vi "Temperature Response.vi"(8 "error in (no error)":errorcluster, 9 "Diagnostics":string, 10 "Sender":string, 11 "Pulse Controller in":refnum<class "Pulse Controller.lvclass">) -> (0 "error out":errorcluster, 3 "Pulse Controller out":refnum<class "Pulse Controller.lvclass">)   [LabVIEW 2024, in "Pulse Controller.lvclass"]
uses:
  Pulse Controller.lvclass
  Pulse Controller.lvclass/Pulse Controller.ctl
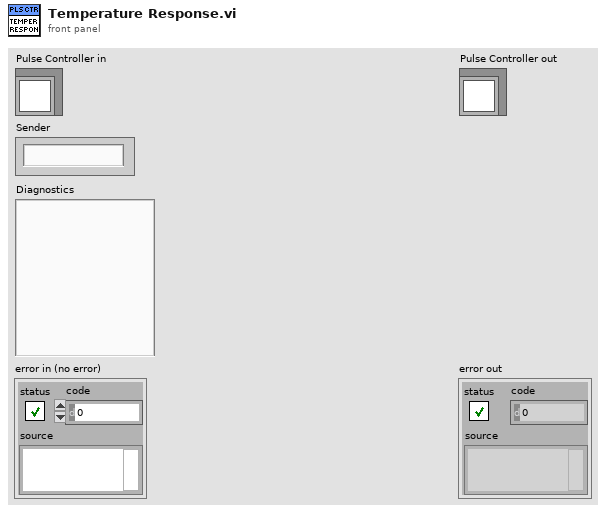
[diagram p1: front panel]
types:
  T1 = typedef "Worker State.ctl" = enum16{"Idle", "Starting", "Working", "Stopping"}
  T2 = cluster{"seconds since 1Jan1904":timestamp, "Sender":string, "Diagnostics":string}
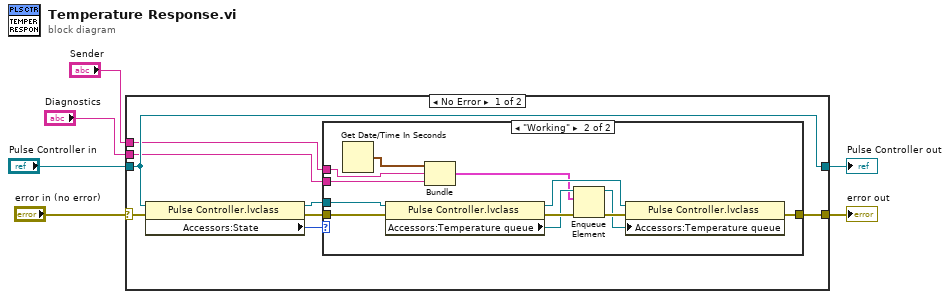
[diagram p0: block diagram]
diagram:
  n1 = case shown="No Error" "error in (no error)" {
    selector: "error in (no error)" -> [w12 w29]
    tunnel: [w11 w29] -> w5
    tunnel: [w14 w28] -> w3
    tunnel: "Pulse Controller in" -> [w14 w28]
    tunnel: "Diagnostics" -> [w9 _]
    tunnel: "Sender" -> [w8 _]
    frame No Error {
      n2 = property class="Pulse Controller.lvclass"(reference=w14, error in=w12) -> (reference out=w7:refnum<class "Pulse Controller.lvclass">, error out=w13:errorcluster, "Accessors:State"=w10:T1)
      n3 = case shown="\"Working\"" w10 {
        tunnel: w13 -> [w15 w23]
        tunnel: [w15 w20] -> w11
        tunnel: w9 -> [_ w26]
        tunnel: w8 -> [_ w25]
        tunnel: w7 -> [_ w24]
        frame "Idle", Default {
        }
        frame "Working" {
          n4 = Get Date/Time In Seconds() -> (seconds since 1Jan1904=w27:timestamp)
          n5 = property class="Pulse Controller.lvclass"(reference=w24, error in=w23) -> (reference out=w19:refnum<class "Pulse Controller.lvclass">, error out=w22:errorcluster, "Accessors:Temperature queue"=w18:refnum<queue>)
          n6 = Bundle("seconds since 1Jan1904"=w27, "Sender"=w25, "Diagnostics"=w26) -> (w17:T2)  [unwired: 1 in]
          n7 = Enqueue Element(queue=w18, element=w17, error in (no error)=w22) -> (queue out=w16:refnum<queue>, error out=w21:errorcluster)  [unwired: 1 in, 1 out]
          n8 = property class="Pulse Controller.lvclass"(reference=w19, error in=w21, "Accessors:Temperature queue"=w16) -> (error out=w20:errorcluster)  [unwired: 1 out]
        }
      }
    }
    frame Error {
    }
  }
  "error out" <- w5
  "Pulse Controller out" <- w3
